vi "Return Code.vi"(8 "error in (no error)":errorcluster, 11 "Return Code":i32) -> (0 "error out":errorcluster, 3 "Return Code Description":u16(ring) items=["Accepted/No Error", "Incorrect Message Format", "Incorrect Message Length", "CRC Error", "Unrecognized Command", "Argument Out of Range", "Argument Parse Error", "Operation Not Permitted", "Operation Failed"])   [LabVIEW 2016]
panel:
  out "element":string
  out "Strings []":string[](array[string])
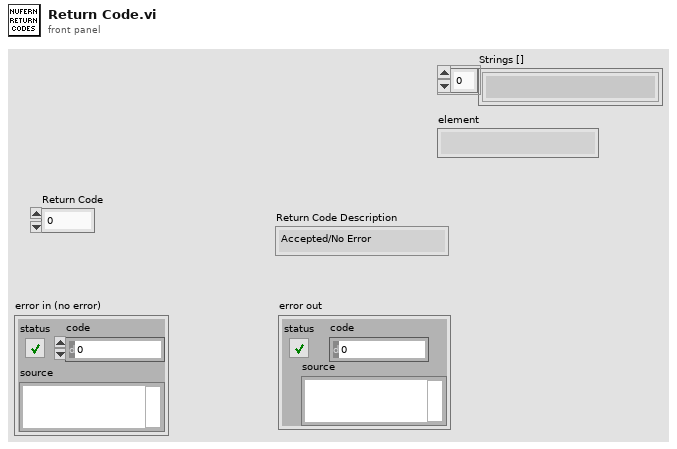
[diagram p1: front panel]
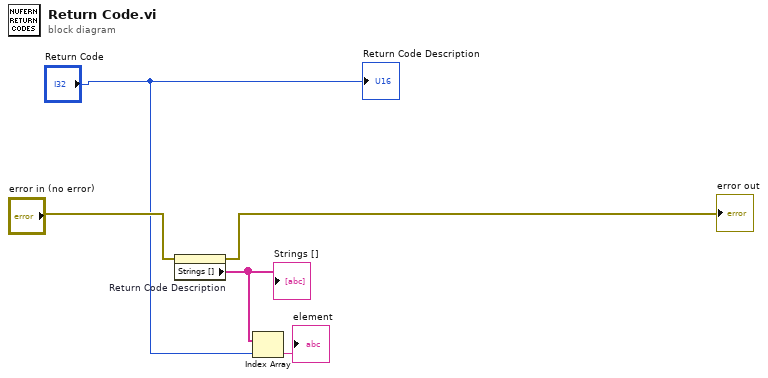
[diagram p0: block diagram]
diagram:
  n1 = property on="Return Code Description" class="Ring (strict)"(error in="error in (no error)") -> (error out=→"error out":errorcluster, "Strings []"=w3:string[])  [unwired: 1 in, 1 out]
  "Strings []" <- w3
  n2 = Index Array(array=w3, index="Return Code") -> (element=→"element":string)
  "Return Code Description" <- "Return Code"
